vi "Read Shared Library.vi"(8 "Error In":errorcluster, 11 "SSH In":refnum<class "SSH.lvclass">) -> (0 "Error Out":errorcluster, 2 "libssh2lv Shared Library":path, 3 "SSH Out":refnum<class "SSH.lvclass">)   [LabVIEW 2021, in "Field_RnD_Services_LIBSSH2_Toolkit.lvlib" / "SSH.lvclass"]
doc: "Gets the path to the libssh2lv library."
uses:
  220524-VNA RP FLAT.llb/SSH.lvclass
  220524-VNA RP FLAT.llb/SSH.lvclass/SSH.ctl
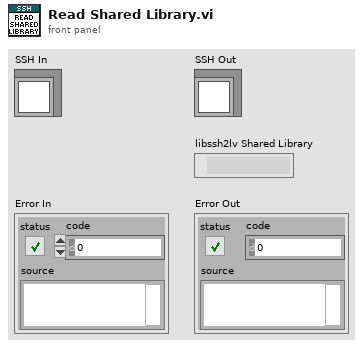
[diagram p1: front panel]
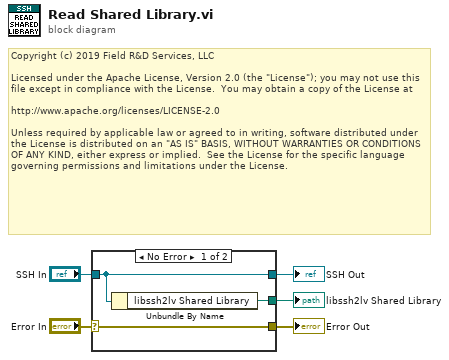
[diagram p0: block diagram]
diagram:
  # "Copyright (c) 2019 Field R&D Services, LLC\n\nLicensed under the Apache License, Version 2.0 (the \"License\"); you may not use this file except in compliance with the License.  You may obtain a copy of the License at\n\nhttp://www.apache.org/licenses/LICENSE-2.0\n\nUnless required by applicable law or agreed to in writing, software distributed under the License is distributed on an \"AS IS\" BASIS, WITHOUT WARRANTIES OR CONDITIONS OF ANY KIND, either express or implied.  See the License for the specific language governing permissions and limitations under the License."
  n1 = case shown="No Error" "Error In" {
    selector: "Error In" -> [w6 w9]
    tunnel: "SSH In" -> [w8 w10]
    tunnel: [w8 w10] -> w3
    tunnel: [w7 _] -> w2
    tunnel: [w6 w9] -> w1
    frame No Error {
      n2 = Unbundle By Name(w8) -> ("libssh2lv Shared Library"=w7:path)
    }
    frame Error {
    }
  }
  "SSH Out" <- w3
  "libssh2lv Shared Library" <- w2
  "Error Out" <- w1
